vi "test.vi"() -> ()   [LabVIEW 2015]
panel:
  out "1-D Array of Real 2":dbl[](array[numeric])
  out "1-D Array of Real":dbl[](array[numeric])
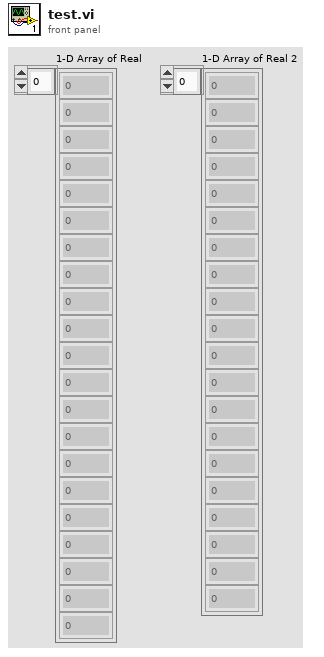
[diagram p1: front panel]
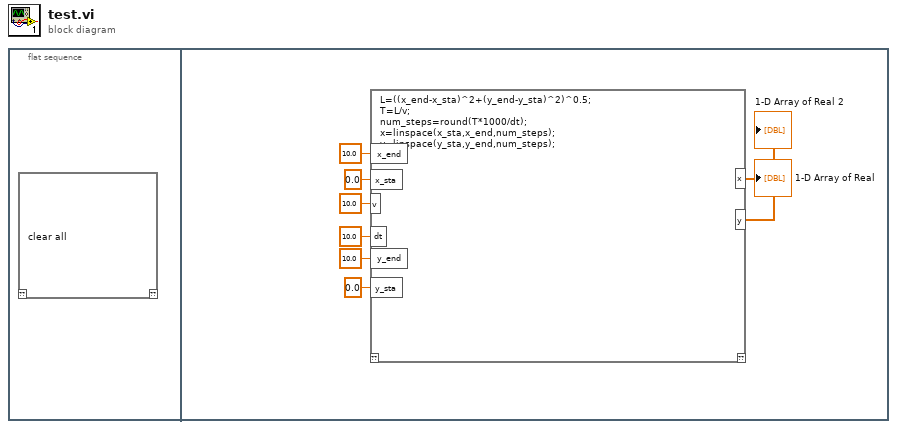
[diagram p0: block diagram]
diagram:
  n1 = flat-sequence {
    frame #0 {
      n2 = script code="clear all"() -> ()  [unwired: 1 in, 1 out]
    }
    frame #1 {
      n3 = script code="L=((x_end-x_sta)^2+(y_end-y_sta)^2)^0.5;\nT=L/v;\nnum_steps=round(T*1000/dt);\nx=linspace(x_sta,x_end,num_steps);\ny=linspace(y_sta,y_end,num_steps);"("x_end"=10.0 ("Real"), "x_sta"=0.0 ("Real"), "v"=10.0 ("Real"), "dt"=10.0 ("Real"), "y_end"=10.0 ("Real"), "y_sta"=0.0 ("Real")) -> ("x"=→"1-D Array of Real":dbl[], "y"=→"1-D Array of Real 2":dbl[])  [unwired: 1 in, 1 out]
    }
  }
